vi "SetTorque(mNm).vi"(8 "error in (no error)":errorcluster, 10 "Torque(mNm)":dbl, 11 "Motor Base in":refnum<class "Motor Base.lvclass">) -> (0 "error out":errorcluster, 3 "Motor Base out":refnum<class "Motor Base.lvclass">)   [LabVIEW 2016, in "Motor Base.lvlib" / "Motor Base.lvclass"]
uses:
  Motor Base.lvclass
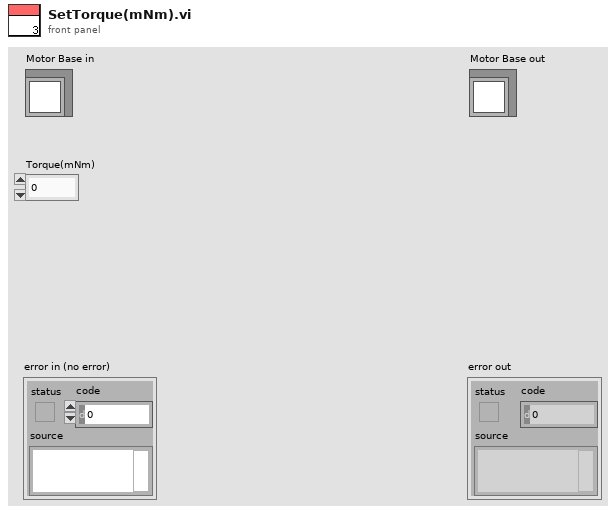
[diagram p1: front panel]
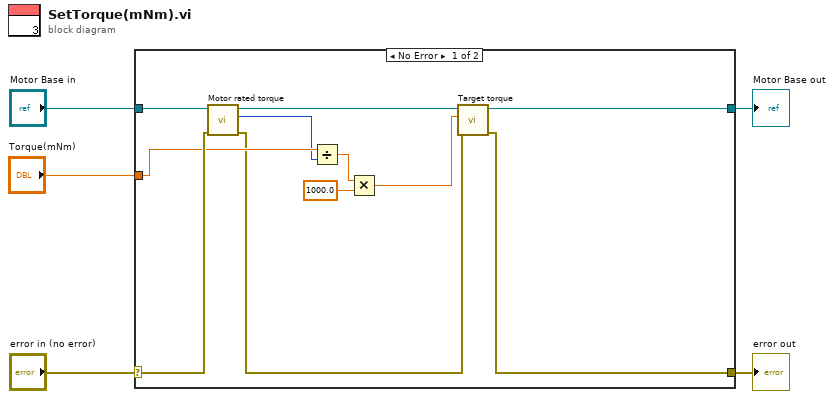
[diagram p0: block diagram]
diagram:
  n1 = case shown="No Error" "error in (no error)" {
    selector: "error in (no error)" -> [w15 w18]
    tunnel: [w7 w18] -> w4
    tunnel: [w6 w17] -> w2
    tunnel: "Motor Base in" -> [w16 w17]
    tunnel: "Torque(mNm)" -> [w14 _]
    frame No Error {
      n2 = call-dynamic "Motor rated torque.vi"("error in"=w15, "Motor Base in"=w16) -> ("error out"=w8:errorcluster, "Data"=w13:u32, "Motor Base out"=w10:refnum<class "Motor Base.lvclass">)  [unwired: 7 in]
      n3 = Divide(x=w14, y=w13) -> (x/y=w12:dbl)
      n4 = Multiply(x=w12, y=1000.0) -> (x*y=w9:dbl)
      n5 = call-dynamic "Target torque.vi"("error in"=w8, "Data"=w9, "Motor Base in"=w10) -> ("error out"=w7:errorcluster, "Motor Base out"=w6:refnum<class "Motor Base.lvclass">)  [unwired: 6 in, 1 out]
    }
    frame Error {
    }
  }
  "error out" <- w4
  "Motor Base out" <- w2
